vi "Auto_Routine_StraightTwoPieceTRAJ.vi"(8 "error in (no error)":errorcluster) -> (0 "error out":errorcluster)   [LabVIEW 2023]
uses:
  Arm2/ArmGetSetpointEnum.ctl
  Trajectory/TrajectoryGlobals.vi
  <vilib>/Rock Robotics/WPI/ThirdParty/JAS_Junk/TrajLib/Trajectory_Library.lvlib
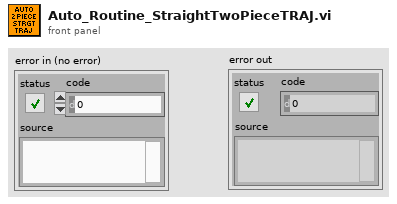
[diagram p1: front panel]
types:
  T1 = typedef "ArmGetSetpointEnum.ctl" = enum16{"ArmFloorPickup", "ArmAmpDeposit", "ArmSpeakerShoot", "ArmStartPosition", "ArmRestPosition", "ArmSourceIntake", "ArmAwayShoot"}
  T2 = typedef "Trajectory_Library.lvlib/TRAJECTORY.ctl" = cluster{"TotalTImeSecs":dbl, "States":T3[]}
  T3 = typedef "Trajectory_Library.lvlib/TRAJ_STATE.ctl" = cluster{"TimeSeconds":dbl, "Velocity":dbl, "Acceleration":dbl, "POSE":T4, "Curvature":dbl}
  T4 = typedef "Trajectory_Library.lvlib/POSE2D.ctl" = cluster{"TRANSLATION":T5, "ROTATION":T6}
  T5 = typedef "Trajectory_Library.lvlib/TRANSLATION2D.ctl" = cluster{"X":dbl, "Y":dbl}
  T6 = typedef "Trajectory_Library.lvlib/ROTATION2D.ctl" = cluster{"VALUE":dbl, "COS":dbl, "SIN":dbl}
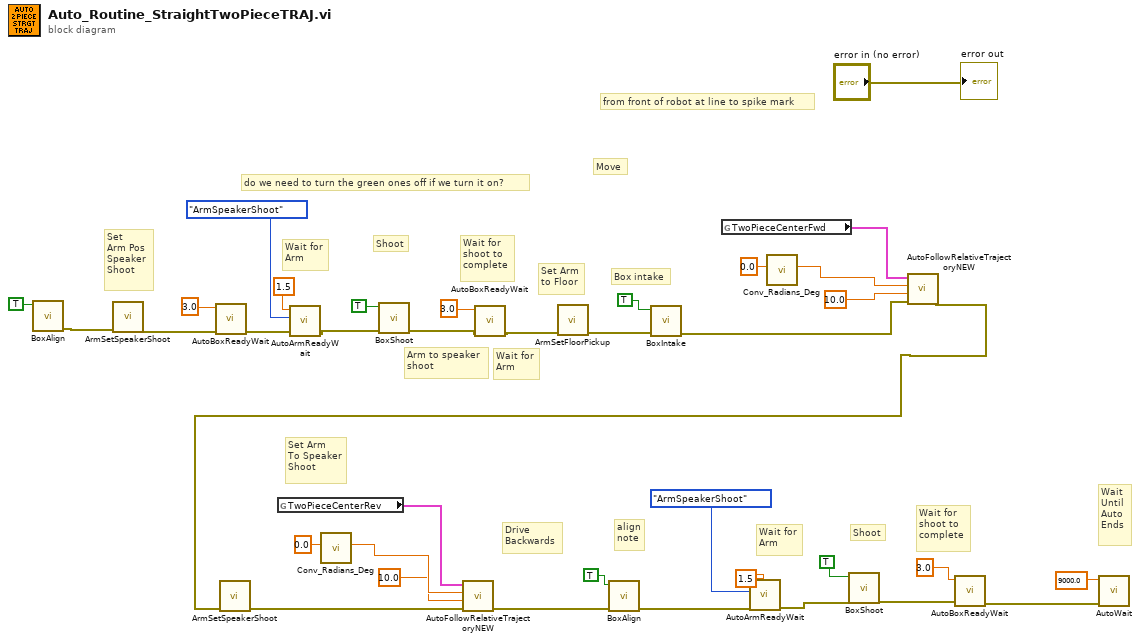
[diagram p0: block diagram]
diagram:
  # "align\nnote"
  # "Wait\nUntil\nAuto \nEnds"
  # "Wait for\nshoot to\ncomplete"
  # "Shoot"
  # "Wait for\nArm"
  # "Drive\nBackwards"
  # "Set Arm\nTo Speaker\nShoot"
  # "Wait for\nArm"
  # "Arm to speaker\nshoot"
  # "Box intake"
  # "Move"
  # "Set Arm\nto Floor"
  # "Wait for\nshoot to\ncomplete"
  # "Shoot"
  # "Wait for\nArm"
  # "Set\nArm Pos\nSpeaker\nShoot"
  # "do we need to turn the green ones off if we turn it on?"
  # "from front of robot at line to spike mark"
  n1 = call "BoxAlign.vi"("box align"=TRUE) -> ("error out"=w20:errorcluster)  [unwired: 10 in]
  n2 = call "ArmSetSpeakerShoot.vi"("error in (no error)"=w20) -> ("error out"=w17:errorcluster)  [unwired: 10 in]
  n3 = call "AutoBoxReadyWait.vi"("error in (no error)"=w17, "TimeOut (s)"=3.0) -> ("error out"=w16:errorcluster)  [unwired: 9 in]
  n4 = global read "TrajectoryGlobals.vi" "TwoPieceCenterRev"() -> (w7:T2)
  n5 = call "AutoArmReadyWait.vi"("error in (no error)"=w16, "ArmSetpoints"=ArmGetSetpointEnum."ArmSpeakerShoot", "TimeOut (s)"=1.5) -> ("error out"=w27:errorcluster)  [unwired: 8 in]
  n6 = call <vilib>:"Conv_Radians_Deg.vi"("Radians"=0.0) -> ("Degrees"=w5:dbl)  [unwired: 10 in]
  n7 = call "BoxShoot.vi"("error in (no error)"=w27, "Box shoot"=TRUE) -> ("error out"=w29:errorcluster)  [unwired: 9 in]
  n8 = call "AutoBoxReadyWait.vi"("error in (no error)"=w29, "TimeOut (s)"=3.0) -> ("error out"=w30:errorcluster)  [unwired: 9 in]
  n9 = call "ArmSetFloorPickup.vi"("error in (no error)"=w30) -> ("error out"=w26:errorcluster)  [unwired: 10 in]
  n10 = call "BoxIntake.vi"("error in (no error)"=w26, "Box intake"=TRUE) -> ("error out"=w9:errorcluster)  [unwired: 9 in]
  n11 = global read "TrajectoryGlobals.vi" "TwoPieceCenterFwd"() -> (w13:T2)
  n12 = call <vilib>:"Conv_Radians_Deg.vi"("Radians"=0.0) -> ("Degrees"=w11:dbl)  [unwired: 10 in]
  n13 = call "AutoFollowRelativeTrajectoryNEW.vi"("error in (no error)"=w9, "TimeOut (s)"=10.0, "End Orientation"=w11, "Trajectory"=w13) -> ("error out"=w8:errorcluster)  [unwired: 7 in]
  n14 = call "ArmSetSpeakerShoot.vi"("error in (no error)"=w8) -> ("error out"=w3:errorcluster)  [unwired: 10 in]
  n15 = call "AutoFollowRelativeTrajectoryNEW.vi"("error in (no error)"=w3, "TimeOut (s)"=10.0, "End Orientation"=w5, "Trajectory"=w7) -> ("error out"=w2:errorcluster)  [unwired: 7 in]
  n16 = call "BoxAlign.vi"("error in (no error)"=w2, "box align"=TRUE) -> ("error out"=w14:errorcluster)  [unwired: 9 in]
  n17 = call "AutoArmReadyWait.vi"("error in (no error)"=w14, "ArmSetpoints"=ArmGetSetpointEnum."ArmSpeakerShoot", "TimeOut (s)"=1.5) -> ("error out"=w32:errorcluster)  [unwired: 8 in]
  n18 = call "BoxShoot.vi"("error in (no error)"=w32, "Box shoot"=TRUE) -> ("error out"=w36:errorcluster)  [unwired: 9 in]
  n19 = call "AutoBoxReadyWait.vi"("error in (no error)"=w36, "TimeOut (s)"=3.0) -> ("error out"=w1:errorcluster)  [unwired: 9 in]
  n20 = call "AutoWait.vi"("error in (no error)"=w1, "TimeOut (s)"=9000.0) -> ()  [unwired: 9 in, 1 out]
  "error out" <- "error in (no error)"
